vi "python image analysis.vi"(8 "error in (no error)":errorcluster, 11 "Point Grey Camera in":refnum<class "Point Grey Camera.lvclass">) -> (0 "error out":errorcluster, 1 "lineouts":dbl[][](array[numeric]), 2 "return value 2":dbl[](array[numeric]), 3 "return value":u16[][](array[numeric]))   [LabVIEW 2020, in "Point Grey Camera.lvclass"]
uses:
  Point Grey Camera.lvclass
  Point Grey Camera.lvclass/Point Grey Camera.ctl
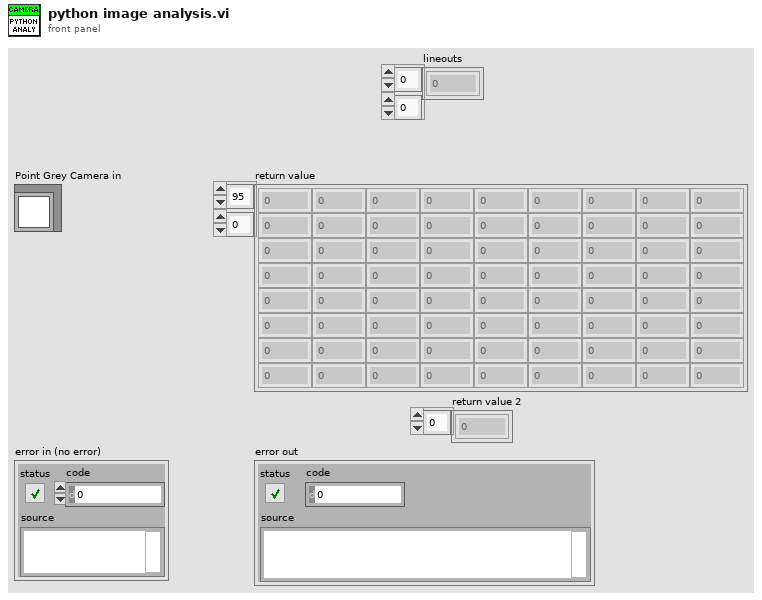
[diagram p1: front panel]
types:
  T1 = cluster{"Processed image":u16[][], "scalar results":dbl[], "lineouts":dbl[][]}
  T2 = typedef "IMAQ Image.ctl" = refnum<image>
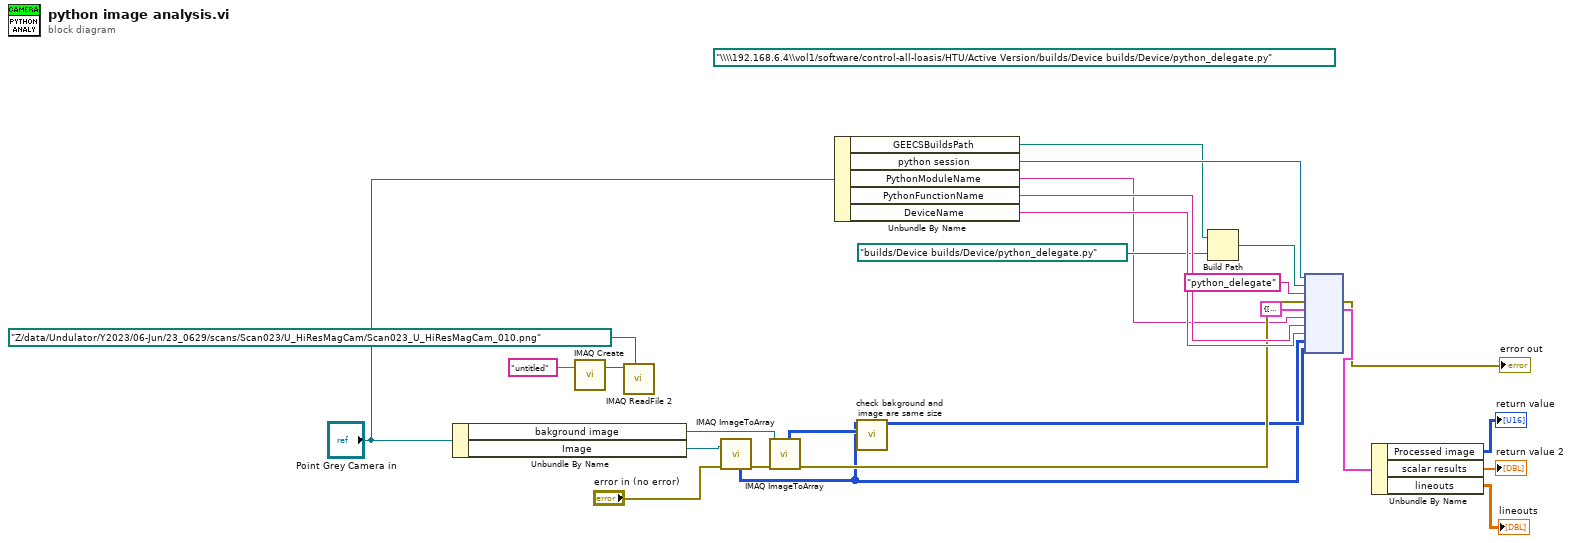
[diagram p0: block diagram]
diagram:
  (unwired) path "\\\\192.168.6.4\\vol1/software/control-all-loasis/HTU/Active Version/builds/Device builds/Device/python_delegate.py" ("module path")
  n1 = Unbundle By Name("Point Grey Camera in") -> ("bakground image"=w2:T2, "Image"=w1:T2)
  n2 = call "IMAQ Create"("Image Name"="untitled") -> ("New Image"=w4:T2)  [unwired: 4 in, 1 out]
  n3 = call "IMAQ ReadFile 2"("File Path"=path "Z:/data/Undulator/Y2023/06-Jun/23_0629/scans/Scan023/U_HiResMagCam/Scan023_U_HiResMagCam_010.png", "Image"=w4) -> ()  [unwired: 5 in, 5 out]
  n4 = call "IMAQ ImageToArray"("error in (no error)"="error in (no error)", "Image"=w1) -> ("Image Pixels (U16)"=w10:u16[][], "error out"=w24:errorcluster)  [unwired: 2 in, 3 out]
  n5 = call "IMAQ ImageToArray"("error in (no error)"=w24, "Image"=w2) -> ("Image Pixels (U16)"=w23:u16[][], "error out"=w12:errorcluster)  [unwired: 2 in, 3 out]
  n6 = Unbundle By Name("Point Grey Camera in") -> ("GEECSBuildsPath"=w9:path, "python session"=w18:refnum<k35>, "PythonModuleName"=w6:string, "PythonFunctionName"=w20:string, "DeviceName"=w21:string)
  n7 = call "check bakground and image are same size.vi"("background array"=w23, "image array"=w10) -> ("background array out"=w11:u16[][])  [unwired: 9 in]
  n8 = Build Path(base path=w9, name or relative path=path "builds/Device builds/Device/python_delegate.py" ("module path")) -> (appended path=w7:path)
  n9 = node(w18, w7, "python_delegate" ("function name"), w12, T1 {"Processed image"=[], "scalar results"=[], "lineouts"=[]}, w6, w20, w21, w10, w11) -> (→"error out":errorcluster, w14:T1)  [unwired: 5 in, 3 out]
  n10 = Unbundle By Name(w14) -> ("Processed image"=→"return value":u16[][], "scalar results"=→"return value 2":dbl[], "lineouts"=→"lineouts":dbl[][])
